vi "Get Settings.vi"(10 "id":string, 11 "DSF Configuration in":T2) -> (0 "exists?":bool, 2 "info":T1, 3 "DSF Configuration out":T2, 4 "index":i32)   [LabVIEW 2017, in "DSF Core.lvlib" / "Configuration Session.lvclass"]
uses:
  Configuration Session.lvclass
  DSF Config Data.ctl
  Internal DSF Configuration.ctl
  Typedefs/DSF Version Info.ctl
  Internal DSF Plugin with ID.ctl
  Internal DSF Plugin Info.ctl
  Typedefs/DSF Timing Info.ctl
  Typedefs/DSF Engine Plugin Thread Configuration.ctl
  Typedefs/DSF Settings Info.ctl
  Internal DSF Group with ID.ctl
  Internal DSF Group Info.ctl
  Internal DSF Transfer with ID.ctl
  Internal DSF Transfer Info.ctl
  Internal DSF Channel with ID.ctl
  Internal DSF Channel Info.ctl
  Internal DSF Settings with ID.ctl
  Internal DSF Settings Info.ctl
  DSF Core.lvlib
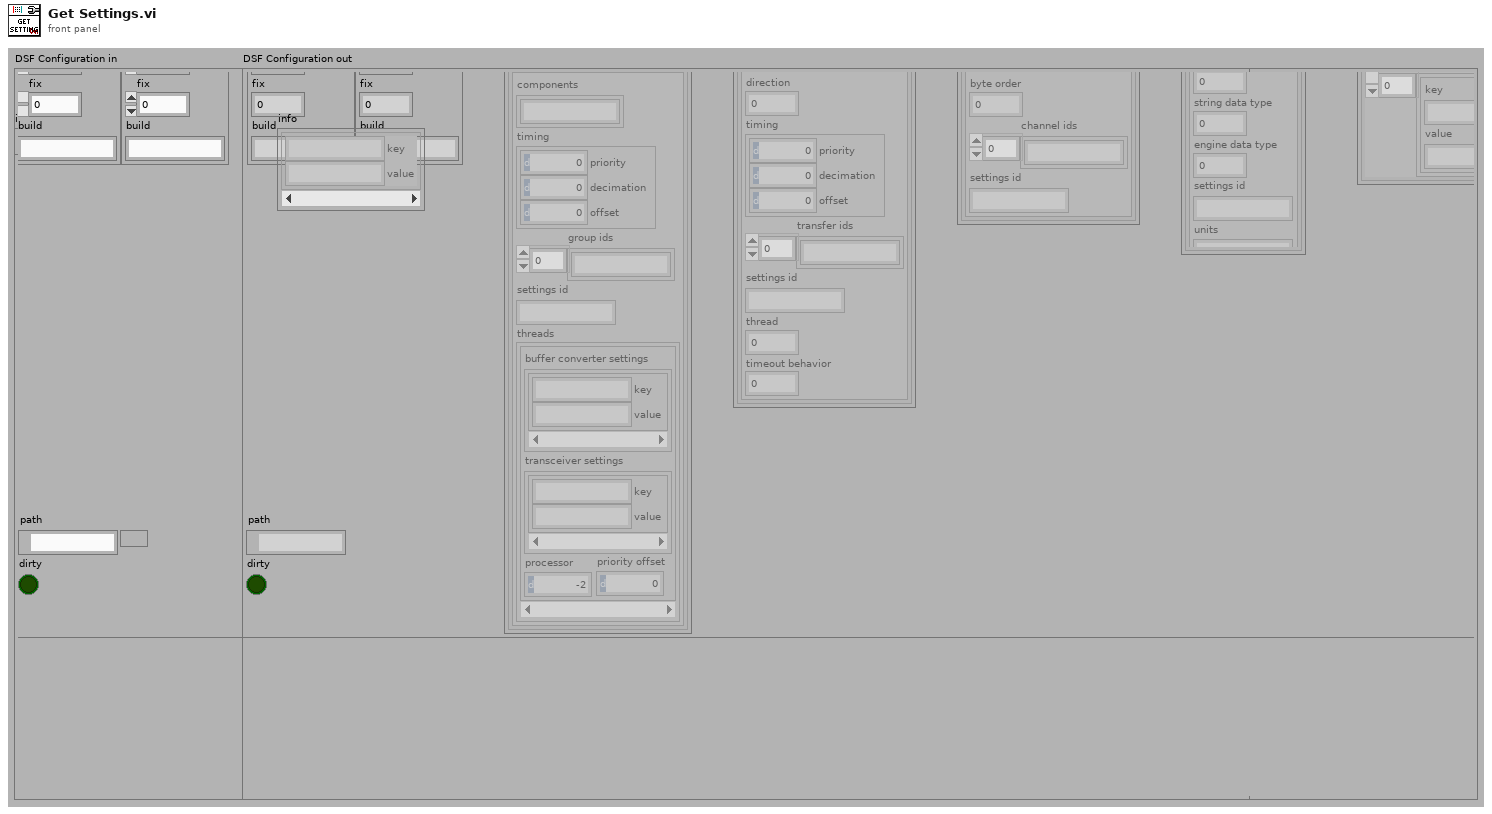
[diagram p1: front panel]
types:
  T1 = typedef "DSF Core.lvlib/DSF Settings Info.ctl" = cluster{"key":string, "value":string}[]
  T2 = typedef "DSF Core.lvlib/Configuration Session.lvclass/DSF Config Data.ctl" = cluster{"dsf configuration":T3, "path":path, "dirty":bool}
  T3 = typedef "DSF Core.lvlib/Configuration Session.lvclass/Internal DSF Configuration.ctl" = cluster{"dsfversion":T4, "version":T4, "plugins":T5[], "groups":T9[], "transfers":T11[], "channels":T13[], "settings":T15[]}
  T4 = typedef "DSF Core.lvlib/DSF Version Info.ctl" = cluster{"major":u32, "minor":u32, "fix":u32, "build":string}
  T5 = typedef "DSF Core.lvlib/Configuration Session.lvclass/Internal DSF Plugin with ID.ctl" = cluster{"id":string, "values":T6}
  T6 = typedef "DSF Core.lvlib/Configuration Session.lvclass/Internal DSF Plugin Info.ctl" = cluster{"components":string[], "timing":T7, "group ids":string[], "settings id":string, "threads":T8[]}
  T7 = typedef "DSF Core.lvlib/DSF Timing Info.ctl" = cluster{"priority":u64, "decimation":u64, "offset":u64}
  T8 = typedef "DSF Core.lvlib/DSF Engine Plugin Thread Configuration.ctl" = cluster{"buffer converter settings":T1, "transceiver settings":T1, "processor":i32, "priority offset":i16}
  T9 = typedef "DSF Core.lvlib/Configuration Session.lvclass/Internal DSF Group with ID.ctl" = cluster{"id":string, "values":T10}
  T10 = typedef "DSF Core.lvlib/Configuration Session.lvclass/Internal DSF Group Info.ctl" = cluster{"direction":i32, "timing":T7, "transfer ids":string[], "settings id":string, "thread":i32, "timeout behavior":u8}
  T11 = typedef "DSF Core.lvlib/Configuration Session.lvclass/Internal DSF Transfer with ID.ctl" = cluster{"id":string, "values":T12}
  T12 = typedef "DSF Core.lvlib/Configuration Session.lvclass/Internal DSF Transfer Info.ctl" = cluster{"byte order":i32, "channel ids":string[], "settings id":string}
  T13 = typedef "DSF Core.lvlib/Configuration Session.lvclass/Internal DSF Channel with ID.ctl" = cluster{"id":string, "values":T14}
  T14 = typedef "DSF Core.lvlib/Configuration Session.lvclass/Internal DSF Channel Info.ctl" = cluster{"string buffer offset":u64, "string data type":i32, "engine data type":i32, "settings id":string, "units":string}
  T15 = typedef "DSF Core.lvlib/Configuration Session.lvclass/Internal DSF Settings with ID.ctl" = cluster{"id":string, "values":T16}
  T16 = typedef "DSF Core.lvlib/Configuration Session.lvclass/Internal DSF Settings Info.ctl" = cluster{"key":string, "value":string}[]
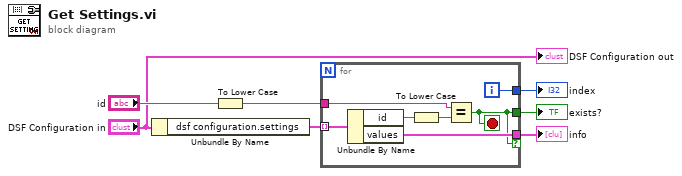
[diagram p0: block diagram]
diagram:
  n1 = Unbundle By Name("DSF Configuration in") -> ("dsf configuration.settings"=w7:T15[])
  n2 = To Lower Case(string="id") -> (all lower case string=w6:string)
  n3 = for {
    tunnel: w7 -> [w14] mode=indexing
    tunnel: w6 -> [w11]
    tunnel: [w8] -> w1
    tunnel: [w10] -> w3
    tunnel: [w9] -> w2 if=w8
    i -> [w10]
    stop <- w8 stop-if-true
    n4 = Unbundle By Name(w14) -> ("id"=w12:string, "values"=w9:T16)
    n5 = To Lower Case(string=w12) -> (all lower case string=w13:string)
    n6 = Equal?(x=w11, y=w13) -> (x = y?=w8:bool)
  }
  "index" <- w3
  "exists?" <- w1
  "info" <- w2
  "DSF Configuration out" <- "DSF Configuration in"
